vi "Example Callback - OzoneConcentration Callback.vi"(4 "OzoneConcentration":refnum<user-event>, 5 "Event Data":T1, 6 "Control Ref":refnum<k24>, 7 "Event Common Data":T2) -> ()   [LabVIEW 2013]
uses:
  C:/tf/play/labview/Tinkerforge.dll
  Tinkerforge.dll
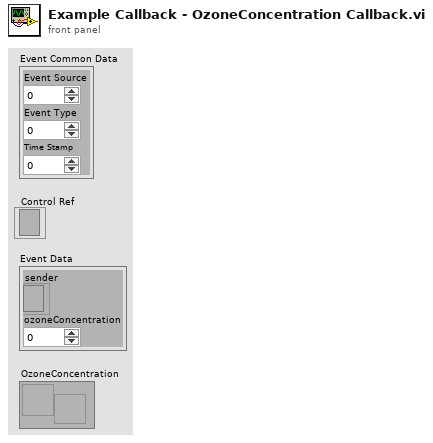
[diagram p1: front panel]
types:
  T1 = cluster{"sender":refnum<k24>, "ozoneConcentration":i32}
  T2 = cluster{"Event Source":i32, "Event Type":u32, "Time Stamp":u32}
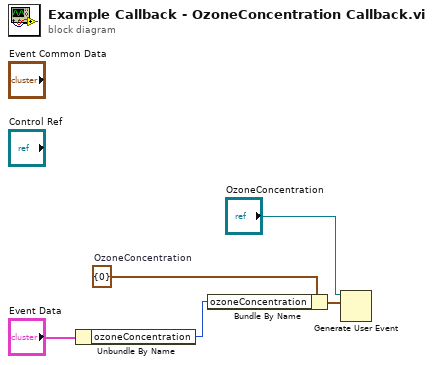
[diagram p0: block diagram]
diagram:
  w3 = cluster{"ozoneConcentration":i32} {"ozoneConcentration"=0}  # OzoneConcentration
  n1 = Unbundle By Name("Event Data") -> ("ozoneConcentration"=w1:i32)
  n2 = Bundle By Name(cluster=w3, "ozoneConcentration"=w1) -> (w4:cluster{"ozoneConcentration":i32})
  n3 = Generate User Event(user event="OzoneConcentration", event data cluster=w4) -> ()  [unwired: 2 in, 2 out]
